vi "Motors Jogger Speed.vi"(5 "Axis Multiplier":u32, 7 "Axis":u32=1, 8 "error in":errorcluster, 9 "VISA in":refnum<visa-resource-name>, 10 "Fast Speed (mm or degree/sec)":dbl, 11 "Normal Speed (mm or degree/sec)":dbl) -> (0 "error out":errorcluster, 1 "VISA out":refnum<visa-resource-name>)   [LabVIEW 2018]
panel:
  out "Read Buffer Fast":string
  out "Read Buffer Normal":string
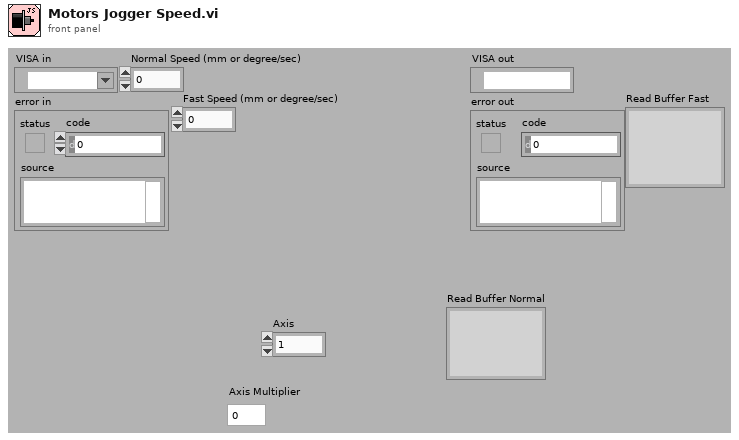
[diagram p1: front panel]
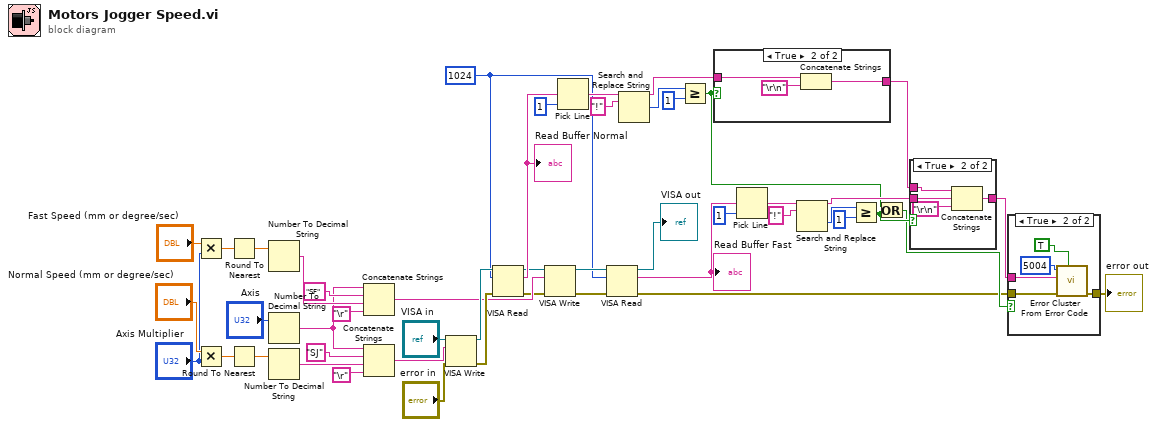
[diagram p0: block diagram]
diagram:
  w21 = 1024
  n1 = Multiply(x="Fast Speed (mm or degree/sec)", y="Axis Multiplier") -> (x*y=w15:dbl)
  n2 = Multiply(x="Normal Speed (mm or degree/sec)", y="Axis Multiplier") -> (x*y=w13:dbl)
  n3 = Round To Nearest(number=w15) -> (nearest integer value=w14:dbl)
  n4 = Round To Nearest(number=w13) -> (nearest integer value=w12:dbl)
  n5 = Number To Decimal String(number=w14) -> (decimal integer string=w35:string)  [unwired: 1 in]
  n6 = Number To Decimal String(number="Axis") -> (decimal integer string=w23:string)  [unwired: 1 in]
  n7 = Number To Decimal String(number=w12) -> (decimal integer string=w42:string)  [unwired: 1 in]
  n8 = Concatenate Strings(w23, "SF", w35, "\r") -> (w34:string)
  n9 = Concatenate Strings(w23, "SJ" ("Command"), w42, "\r") -> (w43:string)
  n10 = VISA Write(VISA resource name="VISA in", write buffer=w43, error in (no error)="error in") -> (VISA resource name out=w46:refnum<visa-resource-name>, error out=w47:errorcluster)  [unwired: 1 out]
  n11 = VISA Read(VISA resource name=w46, byte count=w21, error in (no error)=w47) -> (VISA resource name out=w33:refnum<visa-resource-name>, read buffer=w39:string, error out=w32:errorcluster)  [unwired: 1 out]
  "Read Buffer Normal" <- w39
  n12 = VISA Write(VISA resource name=w33, write buffer=w34, error in (no error)=w32) -> (VISA resource name out=w31:refnum<visa-resource-name>, error out=w30:errorcluster)  [unwired: 1 out]
  n13 = Pick Line(multi-line string=w39, line index=1) -> (output string=w38:string)  [unwired: 1 in]
  n14 = VISA Read(VISA resource name=w31, byte count=w21, error in (no error)=w30) -> (VISA resource name out=→"VISA out":refnum<visa-resource-name>, read buffer=w27:string, error out=w2:errorcluster)  [unwired: 1 out]
  "Read Buffer Fast" <- w27
  n15 = Search and Replace String(input string=w38, search string="!") -> (result string=w37:string, number of replacements=w40:i32)  [unwired: 6 in, 2 out]
  n16 = Greater Or Equal?(x=w40, y=1) -> (x >= y?=w6:bool)
  n17 = case shown="True" w6 {
    tunnel: w37 -> [_ w51]
    tunnel: [_ w50] -> w25
    frame False {
    }
    frame True {
      n18 = Concatenate Strings(w51, "\r\n") -> (w50:string)
    }
  }
  n19 = Pick Line(multi-line string=w27, line index=1) -> (output string=w29:string)  [unwired: 1 in]
  n20 = Search and Replace String(input string=w29, search string="!") -> (result string=w24:string, offset past replacement=w26:i32)  [unwired: 6 in, 2 out]
  n21 = Greater Or Equal?(x=w26, y=1) -> (x >= y?=w5:bool)
  n22 = Or(x=w6, y=w5) -> (x .or. y?=w4:bool)
  n23 = case shown="True" w5 {
    tunnel: w25 -> [w52 w56]
    tunnel: w24 -> [_ w55]
    tunnel: [w52 w54] -> w1
    frame False {
    }
    frame True {
      n24 = Concatenate Strings(w56, w55, "\r\n") -> (w54:string)
    }
  }
  n25 = case shown="True" w4 {
    tunnel: [w57 w61] -> w3
    tunnel: w2 -> [w57 w62]
    tunnel: w1 -> [_ w59]
    frame False {
    }
    frame True {
      n26 = call <vilib>:"Error Cluster From Error Code.vi"("show call chain? (False)"=TRUE, "error in (no error)"=w62, "error message (\"\")"=w59, "error code (0)"=5004) -> ("error out"=w61:errorcluster)  [unwired: 5 in]
    }
  }
  "error out" <- w3
